vi "ArrDtaNmDispOpt.vi"(8 "error in (no error)":errorcluster caption="entrée d'erreur (pas d'erreur)", 11 "BaseDevice en entrée":refnum<class "BaseDevice.lvclass"> caption="DNL_LabVIEW Object in") -> (0 "error out":errorcluster caption="sortie d'erreur", 2 "ArrDisplayNames":string[](array[string]), 3 "BaseDevice en sortie":refnum<class "BaseDevice.lvclass"> caption="DNL_LabVIEW Object out")   [LabVIEW 2019, in "BaseDevice.lvclass"]
uses:
  BaseDevice.lvclass
  BaseDevice.lvclass/BaseDevice.ctl
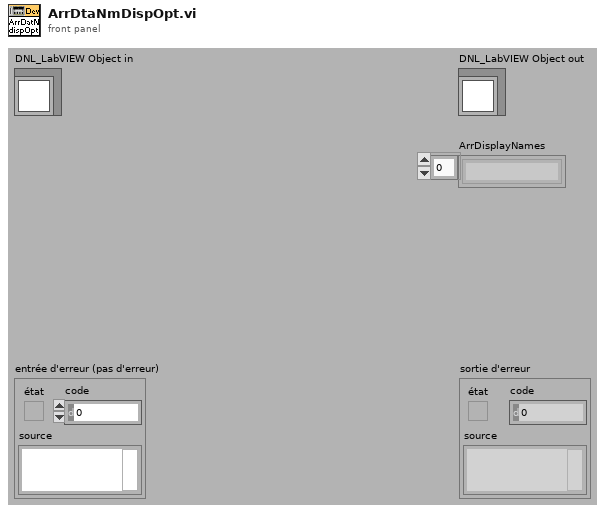
[diagram p1: front panel]
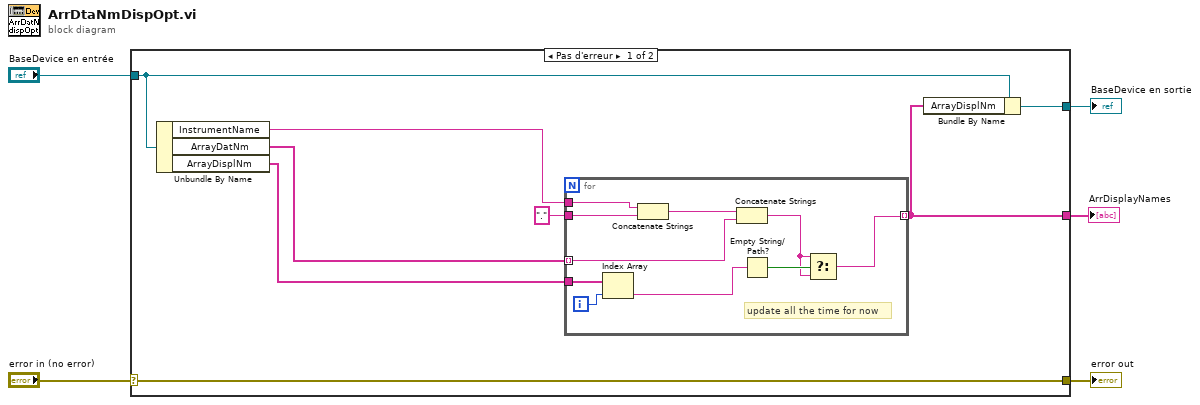
[diagram p0: block diagram]
diagram:
  n1 = case shown="Pas d'erreur" "error in (no error)" {
    selector: "error in (no error)" -> [w13 w25]
    tunnel: [w13 w25] -> w4
    tunnel: [w9 w24] -> w2
    tunnel: "BaseDevice en entrée" -> [w10 w24]
    tunnel: [w8 _] -> w1
    frame No Error {
      n2 = Unbundle By Name(w10) -> ("InstrumentName"=w11:string, "ArrayDatNm"=w6:string[], "ArrayDisplNm"=w7:string[])
      n3 = for {
        tunnel: w6 -> [w17] mode=indexing
        tunnel: w11 -> [w23]
        tunnel: "." ("chaîne") -> [w22]
        tunnel: [w16] -> w8 mode=indexing
        tunnel: w7 -> [w20]
        i -> [w19]
        # "update all the time for now"
        n4 = Index Array(array=w20, index=w19) -> (element=w18:string)
        n5 = Concatenate Strings(w23, w22) -> (w15:string)
        n6 = Concatenate Strings(w15, w17) -> (w14:string)
        n7 = Empty String/Path?(string/path=w18) -> (empty?=w21:bool)
        n8 = Select(t=w14, s=w21, f=w14) -> (s? t:f=w16:string)
      }
      n9 = Bundle By Name(cluster=w10, "ArrayDisplNm"=w8) -> (w9:refnum<class "BaseDevice.lvclass">)
    }
    frame Error {
    }
  }
  "error out" <- w4
  "BaseDevice en sortie" <- w2
  "ArrDisplayNames" <- w1
